vi "Write Process State Data.vi"(8 "error in (no error)":errorcluster, 10 "Process State Data":refnum<data-value>, 11 "Laser Controller in":refnum<class "Laser Controller.lvclass">) -> (0 "error out":errorcluster, 3 "Laser Controller out":refnum<class "Laser Controller.lvclass">)   [LabVIEW 2022 SP3, in "Laser Controller.lvclass"]
uses:
  Laser Controller.lvclass
  XY Stage/Process Actor/Process Framework/Process State Data/Process State Data.lvclass
  Laser Controller.lvclass/Laser Controller.ctl
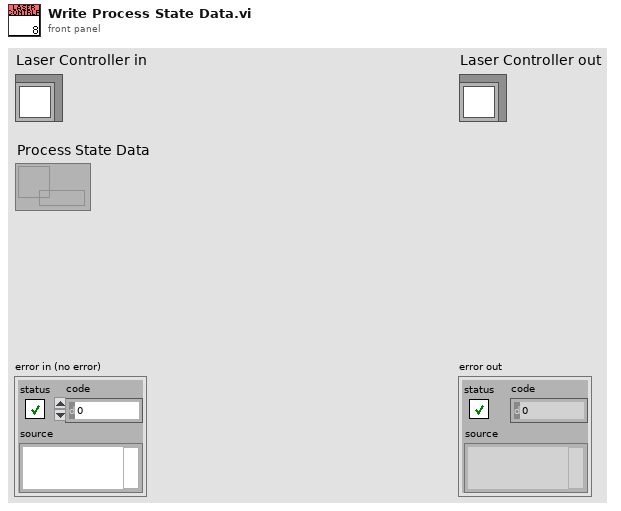
[diagram p1: front panel]
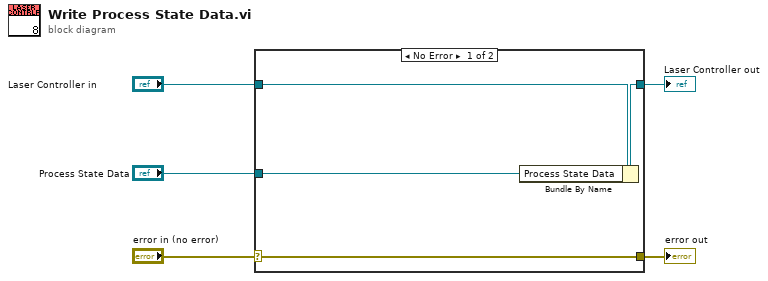
[diagram p0: block diagram]
diagram:
  n1 = case shown="No Error" "error in (no error)" {
    selector: "error in (no error)" -> [w9 w10]
    tunnel: [w9 w10] -> w4
    tunnel: [w7 w11] -> w2
    tunnel: "Laser Controller in" -> [w8 w11]
    tunnel: "Process State Data" -> [w6 _]
    frame No Error {
      n2 = Bundle By Name(cluster=w8, "Process State Data"=w6) -> (w7:refnum<class "Laser Controller.lvclass">)
    }
    frame Error {
    }
  }
  "error out" <- w4
  "Laser Controller out" <- w2
